vi "VIPM_Find Identification Paths.vi"(11 "Filtered map in":map{string, string[]}(c390)) -> (3 "Found Identification Paths":string[](array[string]))   [LabVIEW 2019, in "Project.Dependencies Finder.lvlib" / "Dependency Source_VIPM.lvclass"]
doc: "Find common paths that might be used to identify the package."
uses:
  Dependency Source_VIPM.lvclass
  c2651495-7d7b-4c17-8efa-e050e1766856.vi
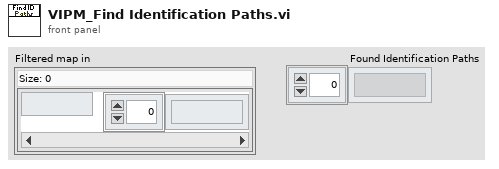
[diagram p1: front panel]
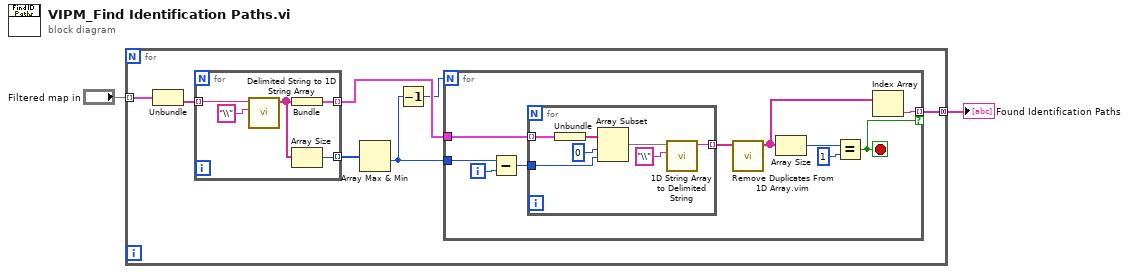
[diagram p0: block diagram]
diagram:
  n1 = for {
    tunnel: "Filtered map in" -> [w9] mode=indexing
    tunnel: [w4] -> w2 mode=concatenating
    n2 = Unbundle(w9) -> ("value"=w8:string[])  [unwired: 1 out]
    n3 = for {
      tunnel: w8 -> [w30] mode=indexing
      tunnel: [w29] -> w7 mode=indexing
      tunnel: [w27] -> w6 mode=indexing
      n4 = call <vilib>:"Delimited String to 1D String Array.vi"("delimiter"="\\" ("search string"), "delimited string"=w30) -> ("string array"=w28:string[])  [unwired: 9 in]
      n5 = Bundle("string array"=w28) -> (w27:cluster{"string array":string[]})  [unwired: 1 in]
      n6 = Array Size(array=w28) -> (size(s)=w29:i32)
    }
    n7 = Array Max & Min(array=w7) -> (min value=w5:i32)  [unwired: 3 out]
    n8 = Decrement(x=w5) -> (x-1=w3:i32)
    n9 = for {
      N: w3 -> [_]
      tunnel: w6 -> [w19]
      tunnel: w5 -> [w18]
      tunnel: [w10] -> w4 mode=indexing if=w11
      i -> [w17]
      stop <- w11 stop-if-true
      n10 = Subtract(x=w18, y=w17) -> (x-y=w16:i32)
      n11 = for {
        tunnel: w19 -> [w26] mode=indexing
        tunnel: w16 -> [w24]
        tunnel: [w20] -> w15 mode=indexing
        n12 = Unbundle(w26) -> ("string array"=w25:string[])
        n13 = Array Subset(array=w25, index=0, length=w24) -> (w23:string[])
        n14 = call <vilib>:"1D String Array to Delimited String.vi"("delimiter"="\\" ("search string"), "string array"=w23) -> ("delimited string"=w20:string)  [unwired: 9 in]
      }
      n15 = call "Remove Duplicates From 1D Array.vim"("array"=w15) -> ("array with duplicates removed"=w12:string[])  [unwired: 10 in]
      n16 = Array Size(array=w12) -> (size(s)=w14:i32)
      n17 = Equal?(x=w14, y=1) -> (x = y?=w11:bool)
      n18 = Index Array(array=w12) -> (element=w10:string)  [unwired: 1 in]
    }
  }
  "Found Identification Paths" <- w2
